vi "Read PIDs from Config.vi"(8 "error in (no error)":errorcluster, 10 "keys":string[](array[string]), 11 "Settings":variant) -> (0 "error out":errorcluster, 2 "Array":T1[](array[typedef]), 3 "Settings out":variant)   [LabVIEW 2018, in "Elevator.lvlib" / "Elevator.lvclass"]
doc: "This VI reads the PIDF values from the configuration file and returns an array of the PIDF's requested from the specific variant."
uses:
  Elevator.lvclass
  <vilib>/Rock Robotics/WPI/ThirdParty/Phoenix-LabVIEW/Motor Controller/Controls/CTRE_Phoenix_MotorControl_SlotStructure.ctl
  b48d7f6c-fa58-4bfe-b1a2-45ef3862d502.vi
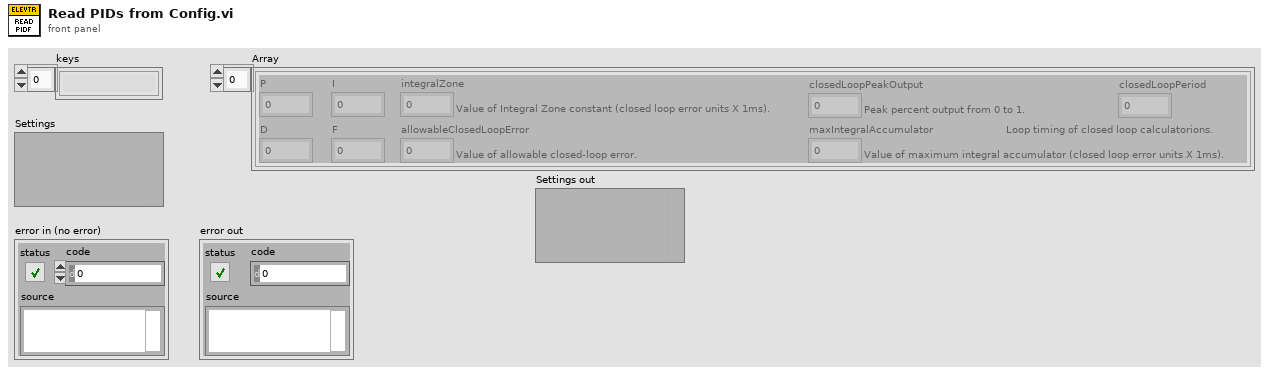
[diagram p1: front panel]
types:
  T1 = typedef "CTRE_Phoenix_MotorControl_SlotStructure.ctl" = cluster{"P":dbl, "I":dbl, "D":dbl, "F":dbl, "integralZone":dbl, "allowableClosedLoopError":i32, "maxIntegralAccumulator":dbl, "closedLoopPeakOutput":dbl, "closedLoopPeriod":i32}
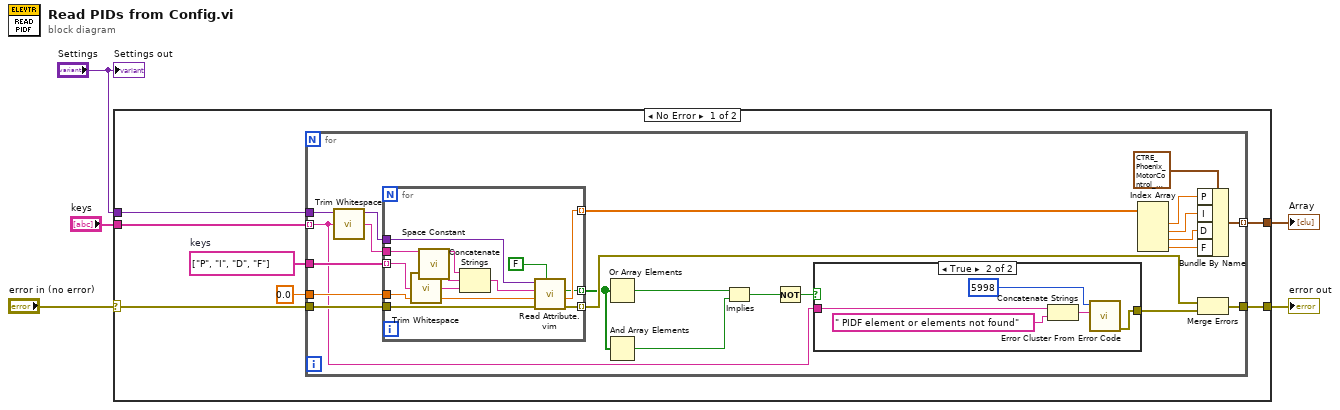
[diagram p0: block diagram]
diagram:
  n1 = case shown="No Error" "error in (no error)" {
    selector: "error in (no error)" -> [w11 w51]
    tunnel: [w6 w51] -> w5
    tunnel: "keys" -> [w10 _]
    tunnel: "Settings" -> [w9 _]
    tunnel: [w7 _] -> w1
    frame No Error {
      w8 = string[] ["P", "I", "D", "F"]  # keys
      n2 = for {
        tunnel: w9 -> [w33]
        tunnel: w10 -> [w13] mode=indexing
        tunnel: w11 -> [w32]
        tunnel: [w16] -> w6
        tunnel: 0.0 -> [w30]
        tunnel: w8 -> [w29]
        tunnel: [w21] -> w7 mode=indexing
        n3 = call <vilib>:"Trim Whitespace.vi"("string"=w13) -> ("trimmed string"=w28:string)  [unwired: 1 in]
        n4 = for {
          tunnel: [w50] -> w22 mode=indexing
          tunnel: w33 -> [w49]
          tunnel: w32 -> [w46]
          tunnel: [w45] -> w31 mode=indexing
          tunnel: w30 -> [w44]
          tunnel: w29 -> [w43] mode=indexing
          tunnel: w28 -> [w41]
          tunnel: [w39] -> w17 mode=indexing
          n5 = call <vilib>:"Trim Whitespace.vi"("string"=w43) -> ("trimmed string"=w42:string)  [unwired: 1 in]
          n6 = call <vilib>:"Space Constant.vi"() -> ("String"=w48:string)
          n7 = Concatenate Strings(w41, w48, w42) -> (w47:string)
          n8 = call "Read Attribute.vim"("Error if not found (T)"=FALSE, "error in"=w46, "default value (data type)"=w44, "name"=w47, "variant in"=w49) -> ("error out"=w45:errorcluster, "value"=w50:dbl, "found"=w39:bool)  [unwired: 3 in, 1 out]
        }
        n9 = Or Array Elements(Boolean array=w17) -> (logical OR=w20:bool)
        n10 = And Array Elements(Boolean array=w17) -> (logical AND=w19:bool)
        n11 = Implies(1:w19, 2:w20) -> (0:w18:bool)
        n12 = Not(x=w18) -> (.not. x?=w14:bool)
        n13 = case shown="True" w14 {
          tunnel: [_ w38] -> w15
          tunnel: w13 -> [_ w36]
          frame False {
          }
          frame True {
            n14 = Concatenate Strings(w36, " PIDF element or elements not found" ("error message (\"\")")) -> (w35:string)
            n15 = call <vilib>:"Error Cluster From Error Code.vi"("error message (\"\")"=w35, "error code (0)"=5998) -> ("error out"=w38:errorcluster)  [unwired: 7 in]
          }
        }
        n16 = Index Array(array=w22) -> (element #1=w27:dbl, element #2=w26:dbl, element #3=w25:dbl, element #4=w24:dbl)  [unwired: 4 in]
        n17 = Bundle By Name(cluster=T1 {"P"=0.0, "I"=0.0, "D"=0.0, "F"=0.0, "integralZone"=0.0, "allowableClosedLoopError"=0, "maxIntegralAccumulator"=0.0, "closedLoopPeakOutput"=1.0, "closedLoopPeriod"=1} ("Elevator Wrist PID"), "P"=w27, "I"=w26, "D"=w25, "F"=w24) -> (w21:T1)
        n18 = Merge Errors(w31, w15) -> (w16:errorcluster)
      }
    }
    frame Error {
    }
  }
  "error out" <- w5
  "Array" <- w1
  "Settings out" <- "Settings"
